vi "Initialize.vi"(8 "Error In":errorcluster, 11 "VI Path":path) -> (0 "Error Out":errorcluster, 1 "Executable Configuration":T2, 2 "Data Structures":T1, 3 "Action Queues":T3)   [LabVIEW 2012]
uses:
  ActionQueues.ctl
  UIActionQueueElement.ctl
  UIAction.ctl
  HardwareActionQueueElement.ctl
  HardwareAction.ctl
  LogActionQueueElement.ctl
  LogAction.ctl
  ExecutableConfiguration.ctl
  DataStructures.ctl
  HardwareDisplayData.ctl
  HardwareLogData.ctl
  libs/LV-Utilities/LV-Utilities.lvlib
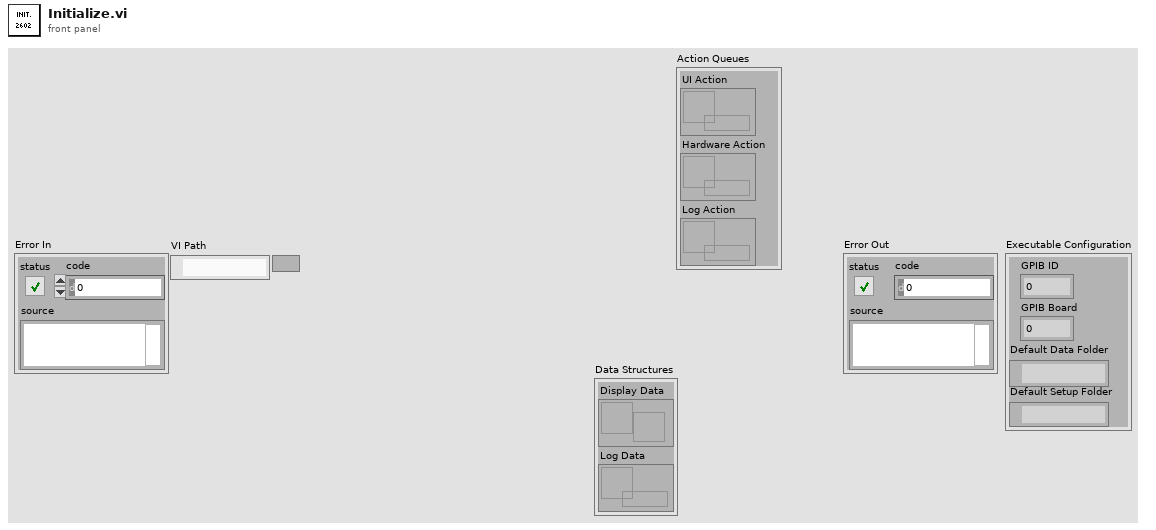
[diagram p1: front panel]
types:
  T1 = typedef "DataStructures.ctl" = cluster{"Display Data":refnum<notifier>, "Log Data":refnum<queue>}
  T2 = typedef "ExecutableConfiguration.ctl" = cluster{"GPIB ID":u8, "GPIB Board":u8, "Default Data Folder":path, "Default Setup Folder":path}
  T3 = typedef "ActionQueues.ctl" = cluster{"UI Action":refnum<queue>, "Hardware Action":refnum<queue>, "Log Action":refnum<queue>}
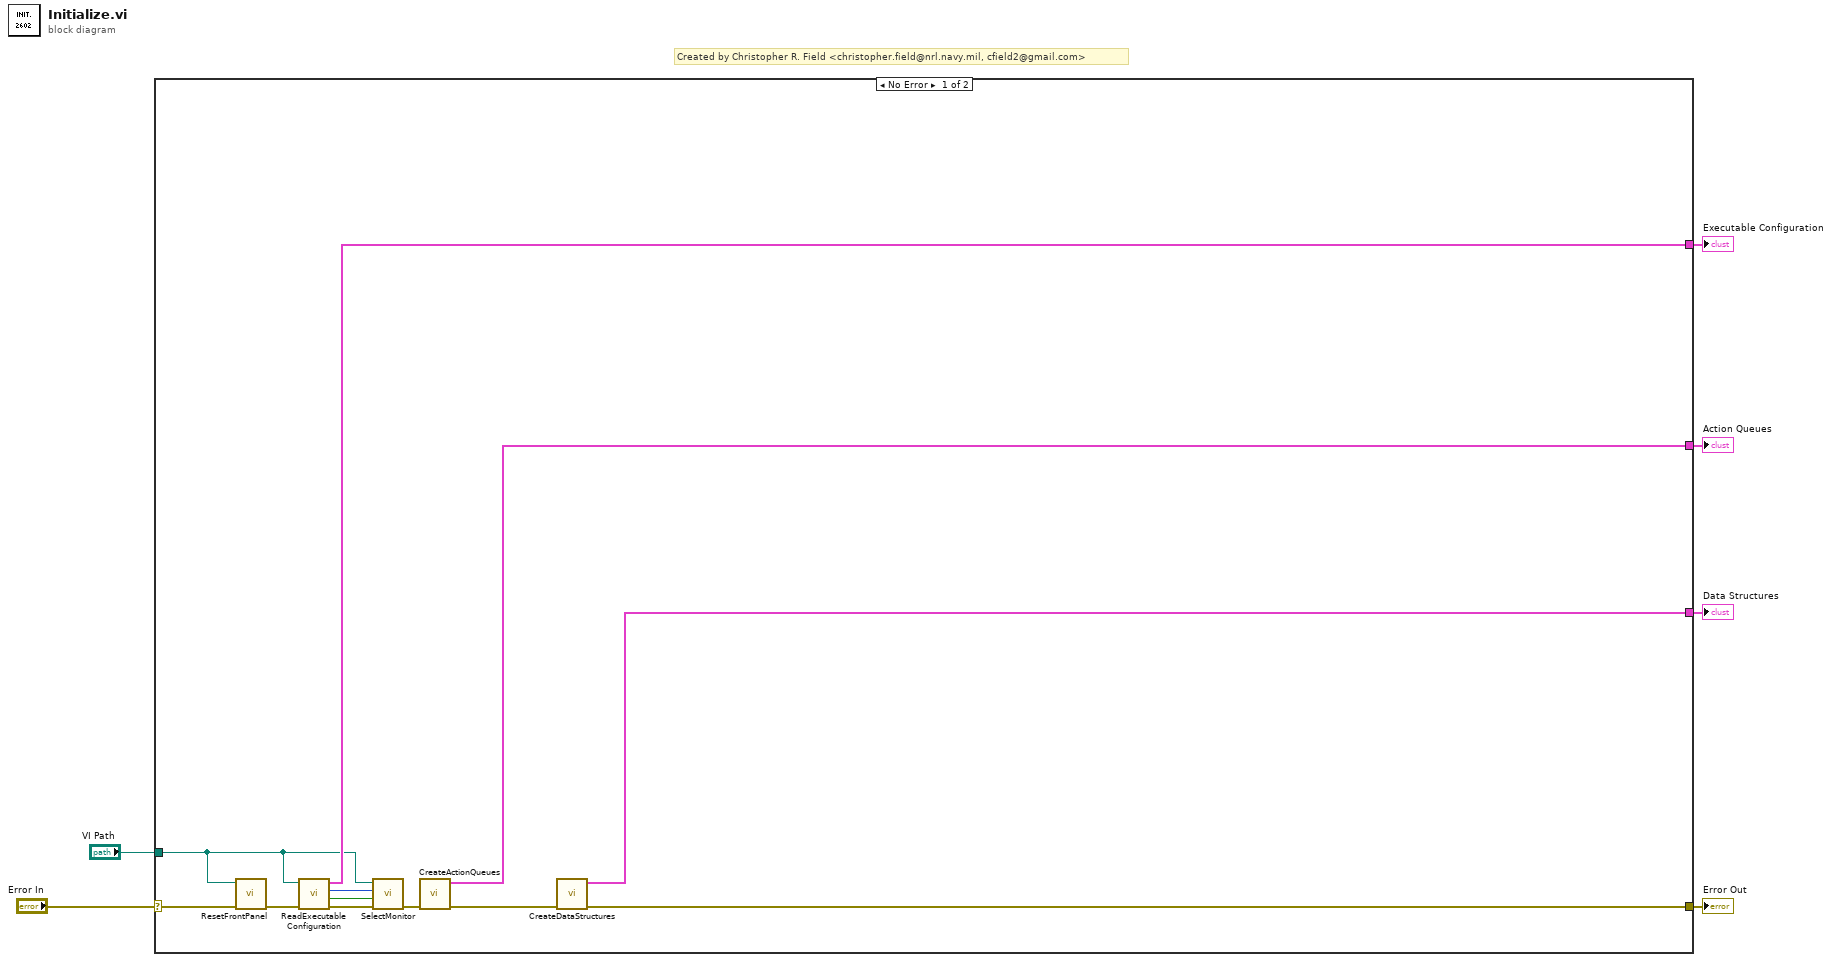
[diagram p0: block diagram]
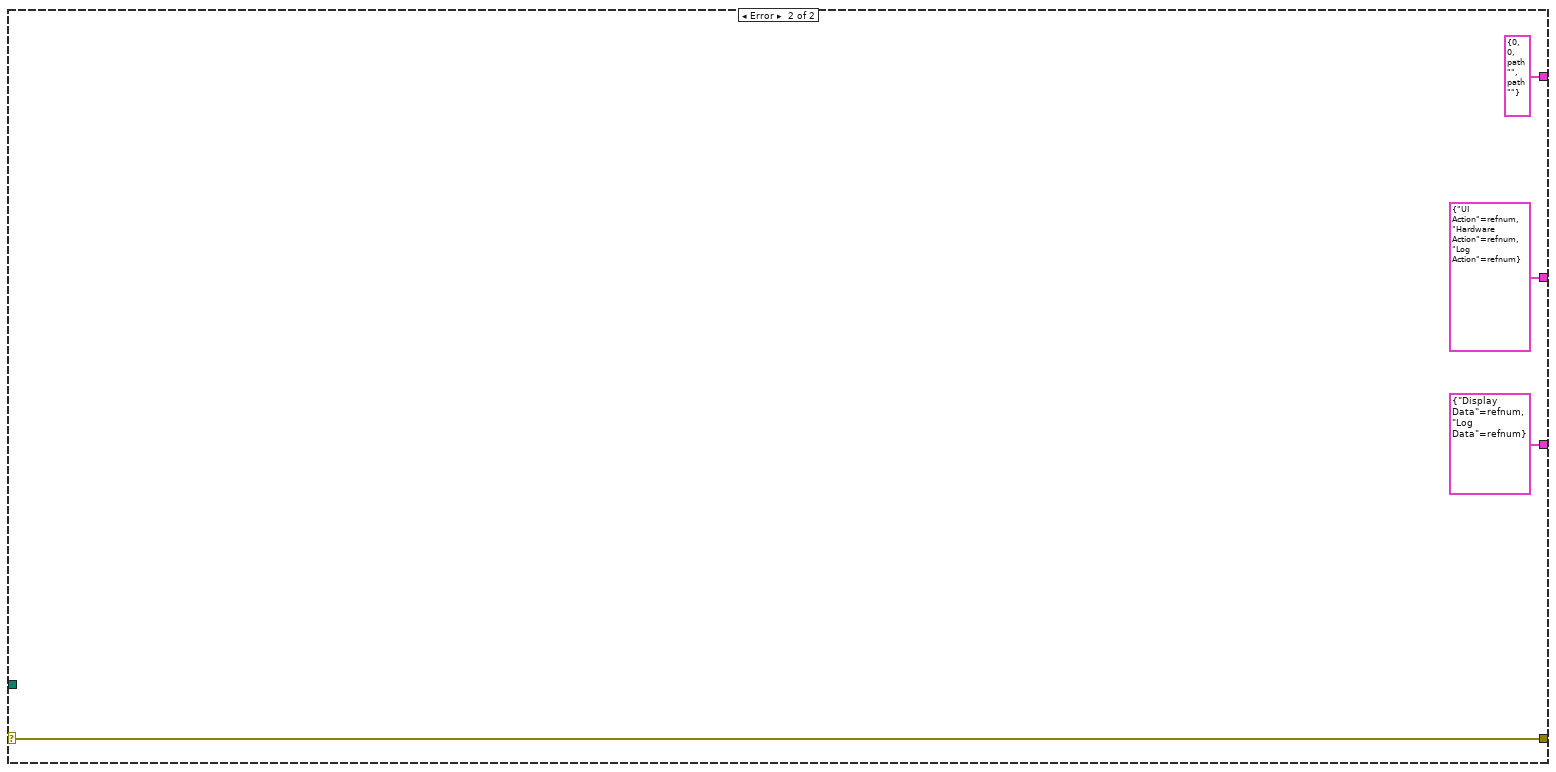
[diagram p2: hidden frame]
diagram:
  # "Created by Christopher R. Field <christopher.field@nrl.navy.mil, cfield2@gmail.com>"
  n1 = case shown="No Error" "Error In" {
    selector: "Error In" -> [w18 w22]
    tunnel: [w10 w22] -> w5
    tunnel: [w16 T3 {"UI Action"=refnum, "Hardware Action"=refnum, "Log Action"=refnum} ("Action Queues")] -> w4
    tunnel: "VI Path" -> [w13 _]
    tunnel: [w14 T2 {"GPIB ID"=0, "GPIB Board"=0, "Default Data Folder"=path "", "Default Setup Folder"=path ""} ("Executable Configuration")] -> w2
    tunnel: [w9 T1 {"Display Data"=refnum, "Log Data"=refnum} ("Data Structures")] -> w1
    frame No Error {
      n2 = call "ResetFrontPanel.vi"("Error In"=w18, "VI Path"=w13) -> ("Error Out"=w15:errorcluster)  [unwired: 9 in]
      n3 = call "ReadExecutableConfiguration.vi"("Error In"=w15, "VI Path"=w13) -> ("Error Out"=w12:errorcluster, "Center on Monitor?"=w7:bool, "Default Monitor"=w8:i32, "Executable Configuration"=w14:T2)  [unwired: 6 in]
      n4 = call "SelectMonitor.vi"("Error In"=w12, "Center?"=w7, "Monitor (0=primary)"=w8, "VI Path"=w13) -> ("Error out"=w17:errorcluster)  [unwired: 7 in]
      n5 = call "CreateActionQueues.vi"("Error In"=w17) -> ("Error Out"=w11:errorcluster, "Action Queues"=w16:T3)  [unwired: 9 in]
      n6 = call "CreateDataStructures.vi"("Error In"=w11) -> ("Error Out"=w10:errorcluster, "Data Structures"=w9:T1)  [unwired: 9 in]
    }
    frame Error {
    }
  }
  "Error Out" <- w5
  "Action Queues" <- w4
  "Executable Configuration" <- w2
  "Data Structures" <- w1
